vi "Test STOMP Connect.vi"() -> ()   [LabVIEW 2017]
uses:
  Typedefs/Type_ServerFrame.ctl
  Typedefs/Type_ServerFrameType.ctl
  STOMP.lvclass
  Typedefs/Type_FrameHeader.ctl
panel:
  out "error out 2":errorcluster
  out "message":T1
  out "error out":errorcluster
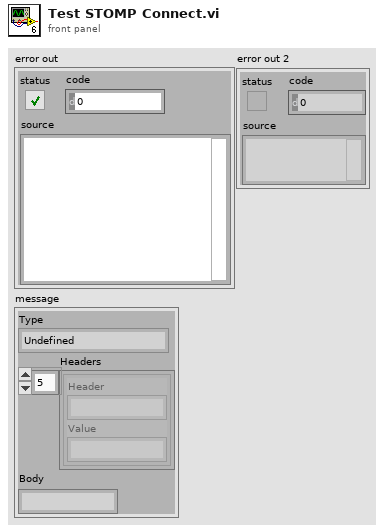
[diagram p1: front panel]
types:
  T1 = typedef "LabVIEW STOMP.lvlib/STOMP.lvclass/Type_ServerFrame.ctl" = cluster{"Type":T2, "Headers":cluster{"Header":string, "Value":string}[], "Body":string}
  T2 = typedef "LabVIEW STOMP.lvlib/STOMP.lvclass/Type_ServerFrameType.ctl" = enum16{"Undefined", "MESSAGE", "CONNECTED", "RECEIPT", "ERROR"}
  T3 = typedef "LabVIEW STOMP.lvlib/STOMP.lvclass/Type_FrameHeader.ctl" = cluster{"Header":string, "Value":string}
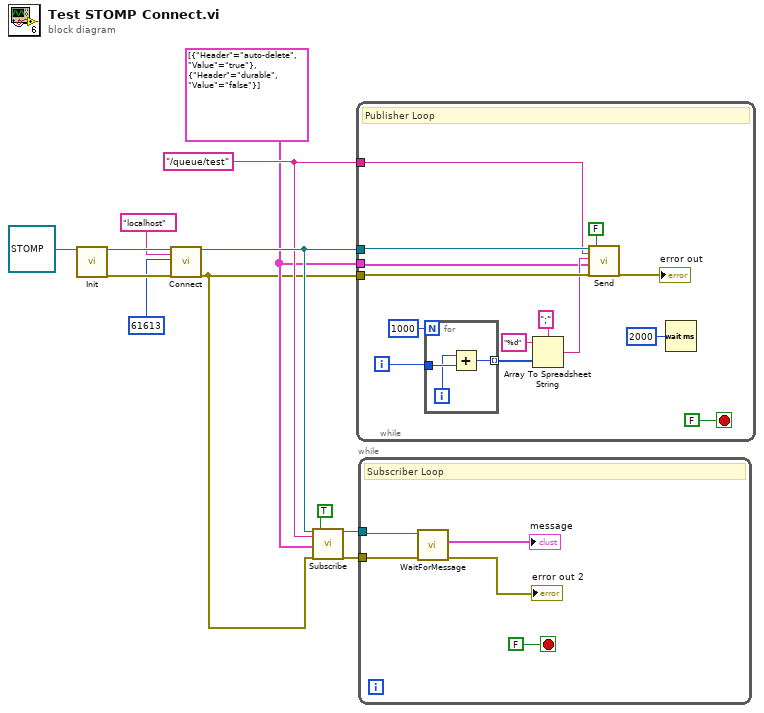
[diagram p0: block diagram]
diagram:
  w2 = T3[] [{"Header"="auto-delete", "Value"="true"}, {"Header"="durable", "Value"="false"}] ("headers")
  w4 = "/queue/test" ("Destination")
  n1 = call "Init.vi"("STOMP in"=refnum<class "STOMP.lvclass"> refnum) -> ("STOMP out"=w11:refnum<class "STOMP.lvclass">, "error out"=w12:errorcluster)  [unwired: 17 in]
  n2 = call "Connect.vi"("STOMP in"=w11, "address"="localhost", "port"=u16 61613, "error in"=w12) -> ("STOMP out"=w7:refnum<class "STOMP.lvclass">, "error out"=w1:errorcluster)  [unwired: 14 in]
  n3 = call-dynamic "Subscribe.vi"("STOMP in"=w7, "Destination"=w4, "headers"=w2, "error in (no error)"=w1, "Receipt?"=TRUE) -> ("STOMP out"=w6:refnum<class "STOMP.lvclass">, "error out"=w5:errorcluster)  [unwired: 13 in]
  n4 = while {
    tunnel: w7 -> [w26]
    tunnel: w4 -> [w21]
    tunnel: w1 -> [w25]
    tunnel: w2 -> [w13]
    i -> [w19]
    stop <- FALSE stop-if-true
    # "Publisher Loop"
    n5 = for {
      N: 1000 -> [_]
      tunnel: w19 -> [w29]
      tunnel: [w27] -> w18 mode=indexing
      i -> [w28]
      n6 = Add(x=w28, y=w29) -> (x+y=w27:i32)
    }
    n7 = Array To Spreadsheet String(delimiter (Tab)=";", array=w18, 3:"%d" ("format string")) -> (spreadsheet string=w14:string)
    n8 = call-dynamic "Send.vi"("STOMP in"=w26, "Destination"=w21, "Body"=w14, "headers"=w13, "error in (no error)"=w25, "Receipt?"=FALSE) -> ("error out"=→"error out":errorcluster)  [unwired: 12 in, 1 out]
    n9 = Wait (ms)(milliseconds to wait=u32 2000) -> ()  [unwired: 1 out]
  }
  n10 = while {
    tunnel: w6 -> [w34]
    tunnel: w5 -> [w33]
    stop <- FALSE stop-if-true
    # "Subscriber Loop"
    n11 = call-dynamic "WaitForMessage.vi"("error in (no error)"=w33, "STOMP in"=w34) -> ("error out"=→"error out 2":errorcluster, "message"=→"message":T1)  [unwired: 7 in, 1 out]
  }
